vi "Mixer.Read Mute.vi"(0 "baseURL":string="http://169.254.128.32/datastore/", 11 "error in (no error)":errorcluster) -> (4 "baseURL out":string="http://169.254.128.32/datastore/", 8 "value":bool, 15 "error out":errorcluster)   [LabVIEW 2020]
uses:
  <vilib>/httpClient/LabVIEWHTTPClient.lvlib
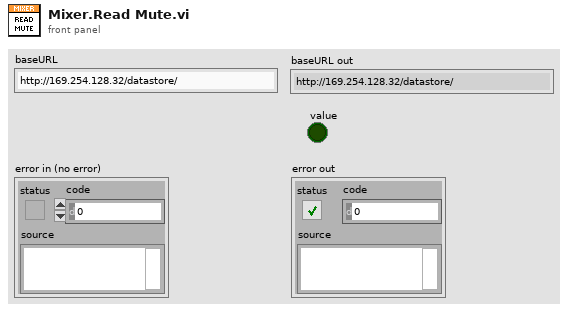
[diagram p1: front panel]
types:
  T1 = typedef "LabVIEWHTTPClient.lvlib/ClientHandle.ctl" = refnum<k1>
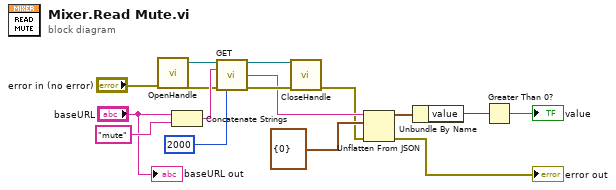
[diagram p0: block diagram]
diagram:
  n1 = call <vilib>:"OpenHandle.vi"("error in (no error)"="error in (no error)") -> ("client handle out"=w12:T1, "error out"=w11:errorcluster)  [unwired: 13 in]
  n2 = Concatenate Strings("baseURL", "mute") -> (w13:string)
  n3 = call <vilib>:"GET.vi"("client handle"=w12, "url"=w13, "error in (no error)"=w11, "timeout (10000)"=2000) -> ("client handle out"=w10:T1, "body"=w8:string, "error out"=w9:errorcluster)  [unwired: 8 in, 1 out]
  n4 = call <vilib>:"CloseHandle.vi"("client handle"=w10, "error in (no error)"=w9) -> ("error out"=w5:errorcluster)  [unwired: 13 in]
  n5 = Unflatten From JSON(JSON string=w8, type and defaults=cluster{"value":i32} {"value"=0}, error in (no error)=w5) -> (value=w6:cluster{"value":i32}, error out=→"error out":errorcluster)  [unwired: 4 in]
  n6 = Unbundle By Name(w6) -> ("value"=w3:i32)
  n7 = Greater Than 0?(x=w3) -> (x > 0?=→"value":bool)
  "baseURL out" <- "baseURL"
